vi "SensorInterrupt.vi"(8 "error in (no error)":errorcluster, 11 "RobotLift in":refnum<class "RobotLift.lvclass">) -> (0 "error out":errorcluster, 3 "RobotLift out":refnum<class "RobotLift.lvclass">)   [LabVIEW 2017, in "RobotLift.lvclass"]
uses:
  RobotLift.lvclass
  Subsystem.lvclass
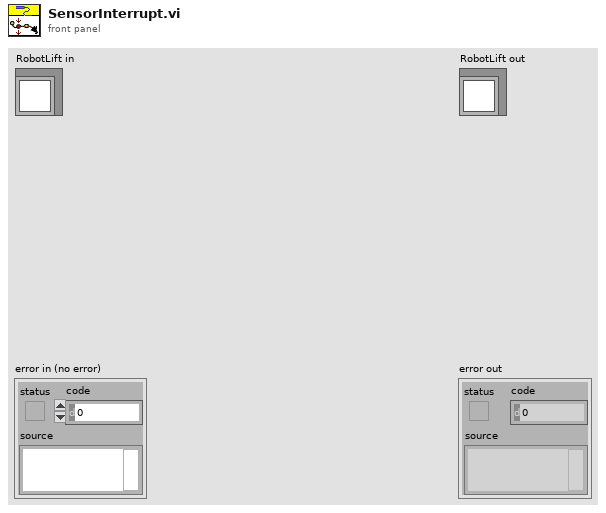
[diagram p1: front panel]
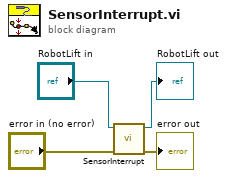
[diagram p0: block diagram]
diagram:
  n1 = call-parent "SensorInterrupt.vi"("error in (no error)"="error in (no error)", "Subsystem in"="RobotLift in") -> ("error out"=→"error out":errorcluster, "Subsystem out"=→"RobotLift out":refnum<class "RobotLift.lvclass">)  [unwired: 8 in]
